vi "jsonConfigToWebsocketConfig.vi"(8 "error in":errorcluster, 10 "StreamCluster_TypeDef":T1={"DAQ"={"ManagmentRate_Hz"=1000, "StreamRate_Hz"=10, "refDesArray"=[], "StreamRate_ms"=0, "ManagmentRate_ms"=1000}, "Modules"=[]}, 11 "jsonConfig":string) -> (0 "error out":errorcluster, 2 "StreamCluster":T1={"DAQ"={"ManagmentRate_Hz"=1000, "StreamRate_Hz"=10, "refDesArray"=[], "StreamRate_ms"=0, "ManagmentRate_ms"=1000}, "Modules"=[]})   [LabVIEW 2024]
uses:
  Control/StreamCluster_TypeDef.ctl
  a79acaf5-1fe2-478e-bd67-a3424b4af532.vi
  e92a0f56-1191-40fe-a6b3-b770361f10d8.vi
  <vilib>/JDP Science/JSONtext/Next JSON Value.vi
  <vilib>/JDP Science/JSONtext/String Subset.vi
  <vilib>/Array/Sort 2D Array - Pop Stack.vi
  <vilib>/Array/Sort 2D Array - Push Stack.vi
  <vilib>/JDP Science/JSONtext/Parsing/Advance past next JSON Value (inlined COPY).vi
  <vilib>/JDP Science/JSONtext/Parsing/Advance past whitespace.vi
  <vilib>/JDP Science/JSONtext/Parsing/Advance past String.vi
  <vilib>/JDP Science/JSONtext/Parsing/Advance past Number.vi
  <vilib>/JDP Science/JSONtext/Parsing/Advance past Line Ending.vi
  <vilib>/JDP Science/JSONtext/Parsing/Parse Full Path or Item Name.vi
  <vilib>/JDP Science/JSONtext/Parsing/Advance past Array.vi
  <vilib>/JDP Science/JSONtext/Parsing/Advance past Object.vi
  <vilib>/JDP Science/JSONtext/support/Error Cluster From Code.vi
  <vilib>/JDP Science/JSONtext/Offset/Find Item Locations by Path.vi
  <vilib>/JDP Science/JSONtext/JSON text to Variant.vi
  <vilib>/JDP Science/JSONtext/LVClass Serializer/JSONtext LVClass Serializer.lvclass
  <vilib>/JDP Science/JSONtext/JSONtext.lvlib
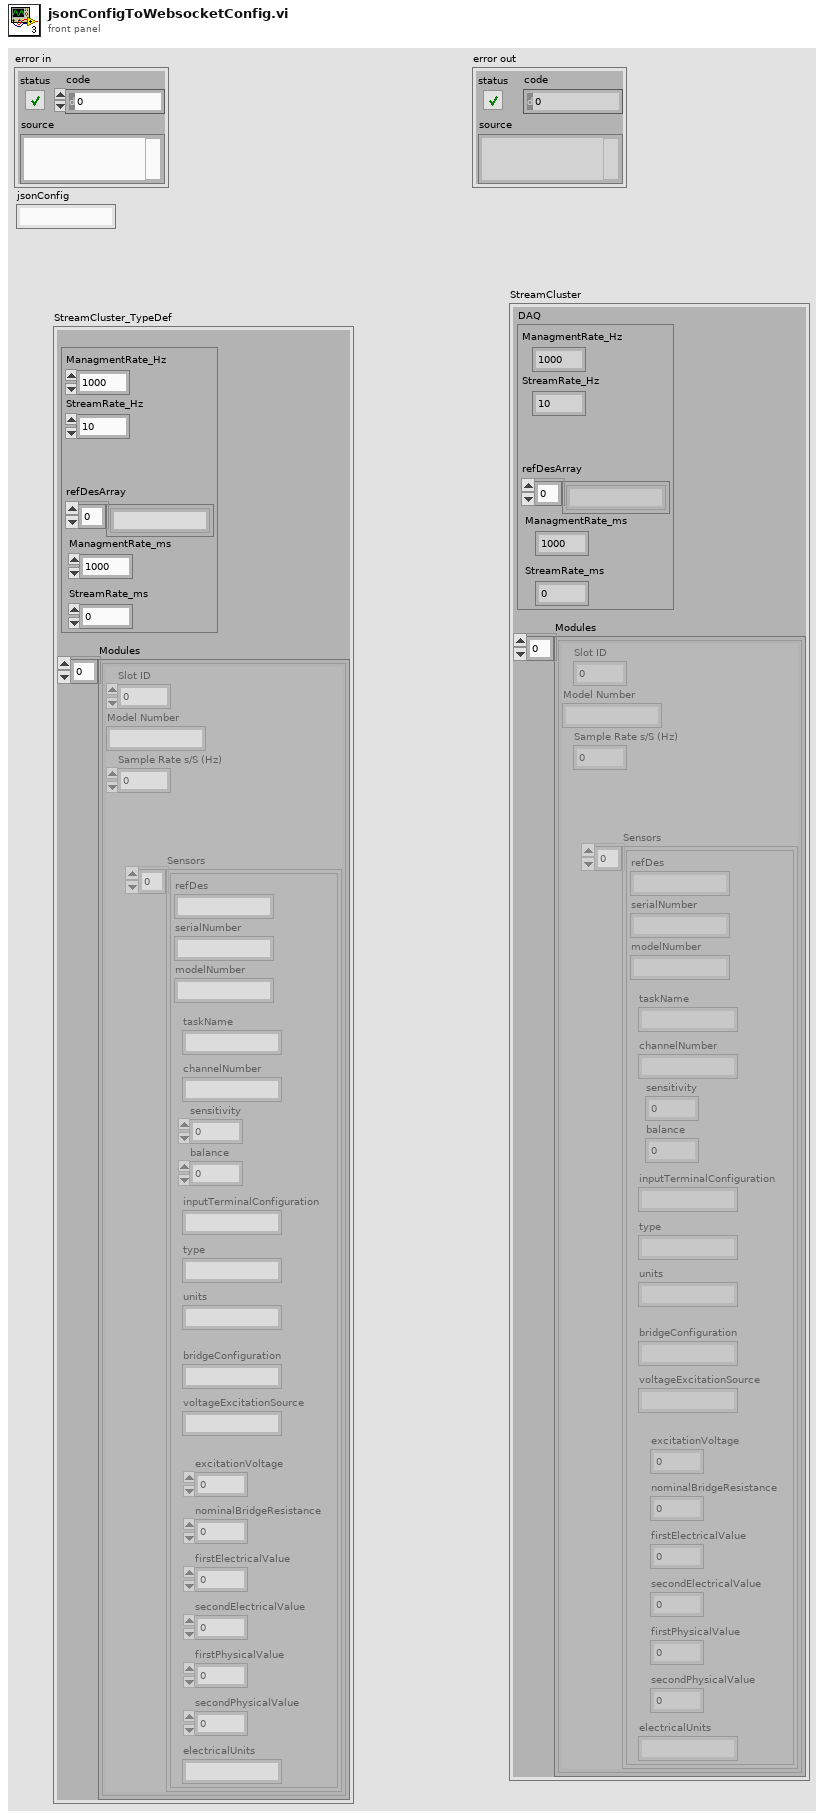
[diagram p1: front panel]
types:
  T1 = typedef "StreamCluster_TypeDef.ctl" = cluster{"DAQ":cluster{"ManagmentRate_Hz":i32, "StreamRate_Hz":i32, "refDesArray":string[], "StreamRate_ms":i32, "ManagmentRate_ms":i32}, "Modules":cluster{"Slot ID":i32, "Model Number":string, "Sample Rate s/S (Hz)":dbl, "Sensors":cluster{"refDes":string, "serialNumber":string, "modelNumber":string, "units":string, "balance":dbl, "sensitivity":dbl, "type":string, "inputTerminalConfiguration":string, "channelNumber":string, "taskName":string, "bridgeConfiguration":string, "excitationVoltage":dbl, "voltageExcitationSource":string, "nominalBridgeResistance":dbl, "firstElectricalValue":dbl, "secondElectricalValue":dbl, "firstPhysicalValue":dbl, "secondPhysicalValue":dbl, "electricalUnits":string}[]}[]}
  T2 = cluster{"[0]":i32, "[1]":i32, "[2]":i32, "[3]":i32, "[4]":i32, "[5]":i32, "[6]":i32, "[7]":i32, "[8]":i32}
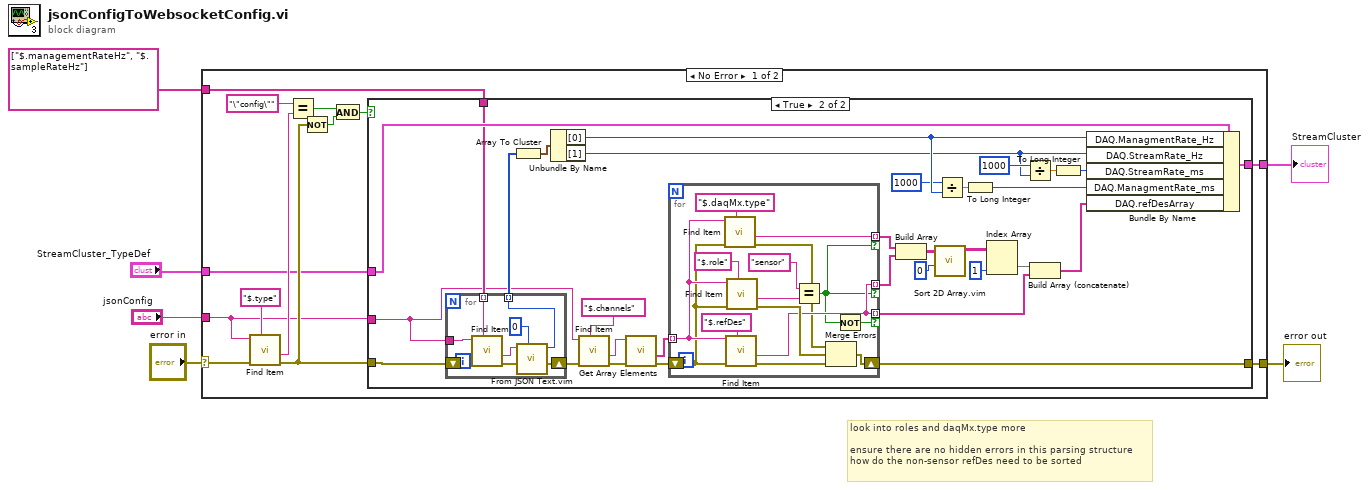
[diagram p0: block diagram]
diagram:
  # "look into roles and daqMx.type more\n\nensure there are no hidden errors in this parsing structure\nhow do the non-sensor refDes need to be sorted"
  n1 = case shown="No Error" "error in" {
    selector: "error in" -> [w12 w77]
    tunnel: [w7 w77] -> w5
    tunnel: "jsonConfig" -> [w10 _]
    tunnel: [w8 w76] -> w3
    tunnel: "StreamCluster_TypeDef" -> [w11 w76]
    tunnel: string[] ["$.managementRateHz", "$.sampleRateHz"] -> [w9 _]
    frame No Error {
      n2 = call <vilib>:"Find Item.vi"("$Path or Item Name"="$.type", "error in (no error)"=w12, "JSON"=w10) -> ("error out"=w19:errorcluster, "<JSON>"=w15:string)  [unwired: 5 in, 2 out]
      n3 = Equal?(x="\"config\"", y=w15) -> (x = y?=w17:bool)
      n4 = Not(x=w19) -> (.not. x?=w18:bool)
      n5 = And(x=w17, y=w18) -> (x .and. y?=w16:bool)
      n6 = case shown="True" w16 {
        tunnel: w19 -> [w20 w50]
        tunnel: w11 -> [w21 w52]
        tunnel: [w21 w51] -> w8
        tunnel: w10 -> [_ w45]
        tunnel: w9 -> [_ w47]
        tunnel: [w20 w40] -> w7
        frame False {
        }
        frame True {
          n7 = for {
            tunnel: w47 -> [w75] mode=indexing
            tunnel: w45 -> [w74]
            tunnel: [w70] -> w49 mode=indexing
            shift-right: [w71] -> w46
            shift-left: w50 -> [w73]
            n8 = call <vilib>:"Find Item.vi"("$Path or Item Name"=w75, "error in (no error)"=w73, "JSON"=w74) -> ("error out"=w72:errorcluster, "<JSON>"=w68:string)  [unwired: 5 in, 2 out]
            n9 = call "From JSON Text.vim"("Data Type and Default Value"=0, "error in (no error)"=w72, "JSON"=w68) -> ("error out"=w71:errorcluster, "Data out"=w70:i32)  [unwired: 7 in]
          }
          n10 = Array To Cluster(array=w49) -> (cluster=w48:T2)
          n11 = Unbundle By Name(w48) -> ("[0]"=w27:i32, "[1]"=w22:i32)
          n12 = call <vilib>:"Find Item.vi"("$Path or Item Name"="$.channels", "error in (no error)"=w46, "JSON"=w45) -> ("error out"=w43:errorcluster, "<JSON>"=w42:string)  [unwired: 5 in, 2 out]
          n13 = call <vilib>:"Get Array Elements.vi"("error in (no error)"=w43, "JSON"=w42) -> ("error out"=w41:errorcluster, "<JSON>"=w39:string[])  [unwired: 7 in, 1 out]
          n14 = for {
            shift-right: [w66] -> w40
            shift-left: w41 -> [w57]
            tunnel: w39 -> [w58] mode=indexing
            tunnel: [w61] -> w31 mode=indexing if=w60
            tunnel: [w61] -> w36 mode=indexing if=w53
            tunnel: [w54] -> w37 mode=indexing if=w53
            n15 = call <vilib>:"Find Item.vi"("$Path or Item Name"="$.daqMx.type", "error in (no error)"=w57, "JSON"=w58) -> ("error out"=w55:errorcluster, "<JSON>"=w54:string)  [unwired: 5 in, 2 out]
            n16 = call <vilib>:"Find Item.vi"("$Path or Item Name"="$.refDes", "error in (no error)"=w57, "JSON"=w58) -> ("error out"=w65:errorcluster, "<JSON>"=w61:string)  [unwired: 5 in, 2 out]
            n17 = call <vilib>:"Find Item.vi"("$Path or Item Name"="$.role", "error in (no error)"=w57, "JSON"=w58) -> ("error out"=w64:errorcluster, "<JSON>"=w62:string)  [unwired: 5 in, 2 out]
            n18 = Equal?(x="sensor", y=w62) -> (x = y?=w53:bool)
            n19 = Merge Errors(w55, w64, w65) -> (w66:errorcluster)
            n20 = Not(x=w53) -> (.not. x?=w60:bool)
          }
          n21 = Build Array(w37, w36) -> (w38:string[][])
          n22 = call "Sort 2D Array.vim"("index"=0, "2D array"=w38) -> ("sorted 2D array"=w34:string[][])  [unwired: 8 in, 1 out]
          n23 = Divide(x=1000, y=w27) -> (x/y=w29:dbl)
          n24 = To Long Integer(number=w29) -> (32bit integer=w28:i32)
          n25 = Index Array(array=w34, index (col)=1) -> (element=w32:string[])  [unwired: 1 in]
          n26 = Divide(x=1000, y=w22) -> (x/y=w24:dbl)
          n27 = Build Array (concatenate)(w32, w31) -> (w30:string[])
          n28 = To Long Integer(number=w24) -> (32bit integer=w23:i32)
          n29 = Bundle By Name(cluster=w52, "DAQ.ManagmentRate_Hz"=w27, "DAQ.StreamRate_Hz"=w22, "DAQ.StreamRate_ms"=w23, "DAQ.ManagmentRate_ms"=w28, "DAQ.refDesArray"=w30) -> (w51:T1)
        }
      }
    }
    frame Error {
    }
  }
  "error out" <- w5
  "StreamCluster" <- w3
